vi "Vision Processing.vi"(4 "error in (no error)":errorcluster, 7 "Image Size":T1=enum."320x240") -> ()   [LabVIEW 2016]
doc: "This VI runs in parallel to other tasks. It gets images from the camera, processes them for color or shape and use that information to affect robot behavior."
uses:
  <vilib>/Rock Robotics/WPI/Camera/WPI_CameraImageSize.ctl
  <vilib>/Rock Robotics/WPI/Camera/WPI_CameraWhite Balance Values.ctl
  <vilib>/Rock Robotics/WPI/Camera/WPI_CameraExposure Values.ctl
  <vilib>/Rock Robotics/WPI/Camera/WPI_CameraFrameRate.ctl
  Robot Global Data.vi
  <vilib>/vision/Image Controls.llb/IMAQ Image.ctl
panel:
  in  "Image Size 2":T1=enum."320x240"
  out "x-y":u32
  out "Gear Data":T2
  out "Peg Data":T2
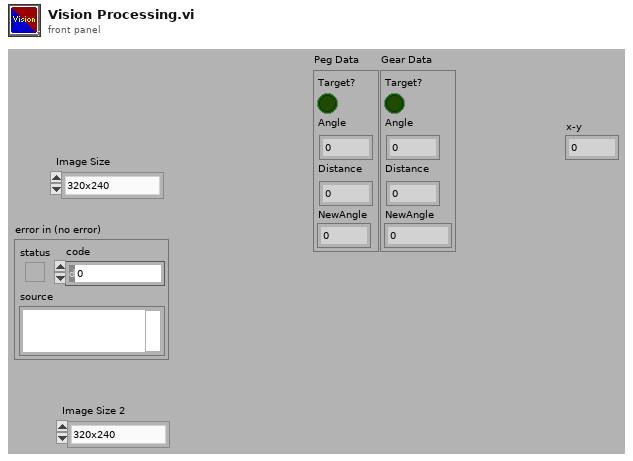
[diagram p1: front panel]
types:
  T1 = typedef "WPI_CameraImageSize.ctl" = enum16{"640x480", "320x240", "160x120", "Custom"}
  T2 = cluster{"Target?":bool, "Angle":dbl, "Distance":dbl, "NewAngle":dbl}
  T3 = typedef "Image Type" = u32
  T4 = typedef "WPI_CameraFrameRate.ctl" = u32
  T5 = typedef "WPI_CameraExposure Values.ctl" = enum16{"Auto", "Flicker-free 50 Hz", "Flicker-free 60 Hz", "Hold current", "Custom"}
  T6 = typedef "WPI_CameraWhite Balance Values.ctl" = enum16{"Auto", "Fixed indoor", "Fixed outdoor 1", "Fixed outdoor 2", "Fixed fluorescent 1", "Fixed fluorescent 2", "Hold current", "Custom"}
  T7 = typedef "IMAQ Image.ctl" = refnum<image>
  T8 = typedef "WPI_CameraDevRef.ctl" = cluster{"Camera Address":string, "CameraStatus":errorcluster}
  T9 = cluster{"Target?":bool, "Angle":dbl, "Distance":dbl}
  T10 = cluster{"Rectangle":cluster{"L":dbl, "T":dbl, "R":dbl, "B":dbl}, "Center":cluster{"X":dbl, "Y":dbl}}
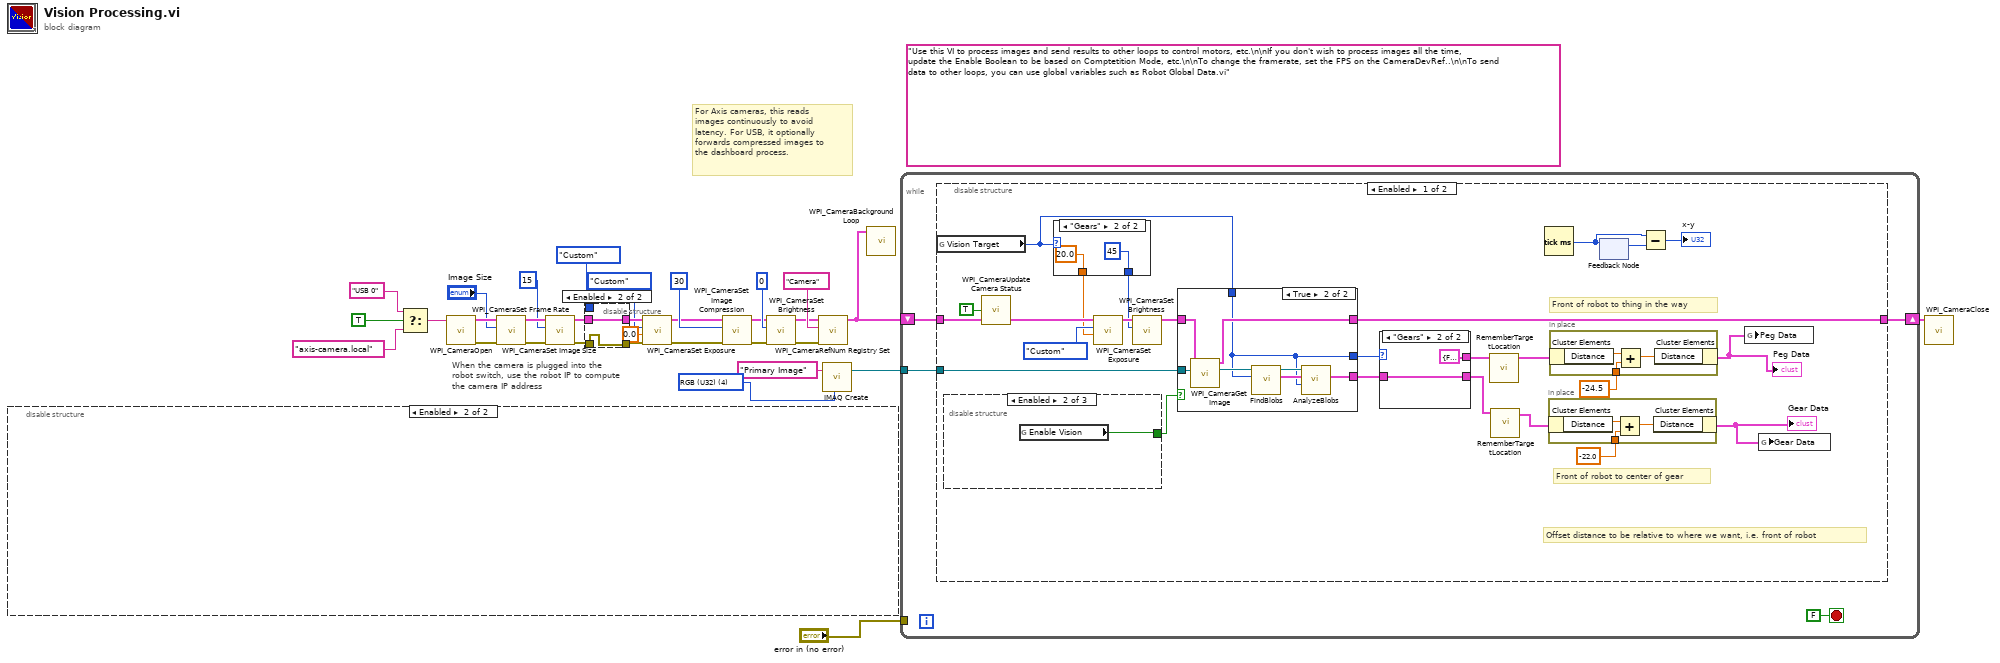
[diagram p0: block diagram]
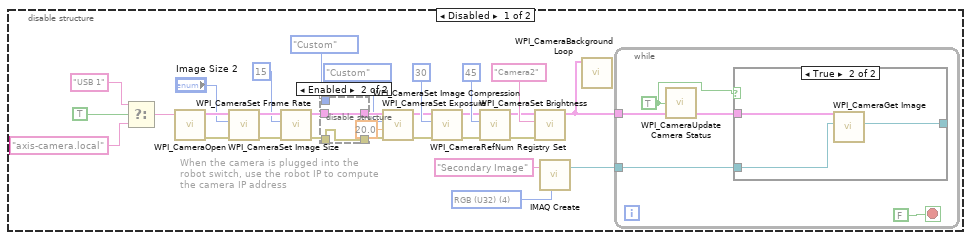
[diagram p2: hidden frame]
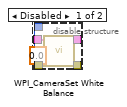
[diagram p3: hidden frame]
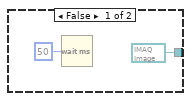
[diagram p4: hidden frame]
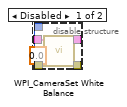
[diagram p5: hidden frame]
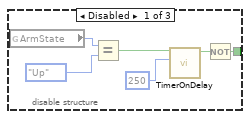
[diagram p6: hidden frame]
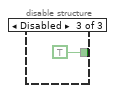
[diagram p7: hidden frame]
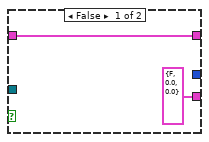
[diagram p8: hidden frame]
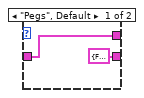
[diagram p9: hidden frame]
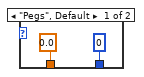
[diagram p10: hidden frame]
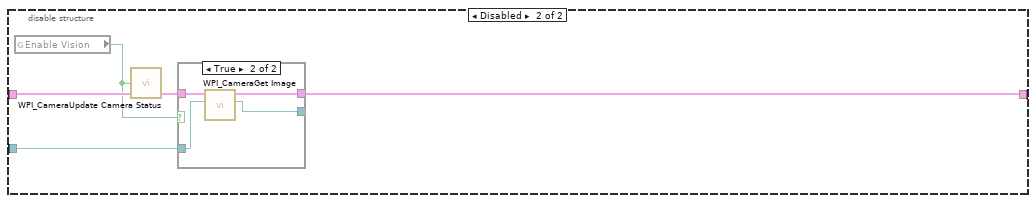
[diagram p11: hidden frame]
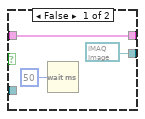
[diagram p12: hidden frame]
diagram:
  w1 = T3 4 items=["Grayscale (U8)", "Grayscale (I16)", "Grayscale (SGL)", "Complex (CSG)", "RGB (U32)", "HSL (U32)", "RGB (U64)"] ("Image Type")
  (unwired) "Use this VI to process images and send results to other loops to control motors, etc.\n\nIf you don't wish to process images all the time, update the Enable Boolean to be based on Comptetition Mode, etc.\n\nTo change the framerate, set the FPS on the CameraDevRef..\n\nTo send data to other loops, you can use global variables such as Robot Global Data.vi"
  # "When the camera is plugged into the\nrobot switch, use the robot IP to compute\nthe camera IP address"
  # "For Axis cameras, this reads\nimages continuously to avoid\nlatency. For USB, it optionally\nforwards compressed images to\nthe dashboard process."
  n1 = disable-structure shown="Enabled" {
    frame Disabled {
      w62 = T3 4 items=["Grayscale (U8)", "Grayscale (I16)", "Grayscale (SGL)", "Complex (CSG)", "RGB (U32)", "HSL (U32)", "RGB (U64)"] ("Image Type")
      # "When the camera is plugged into the\nrobot switch, use the robot IP to compute\nthe camera IP address"
      n2 = Select(t="USB 1" ("format string"), s=TRUE ("dot notation? (F)"), f="axis-camera.local" ("format string")) -> (s? t:f=w37:string)
      n3 = call <vilib>:"WPI_CameraOpen.vi"("Camera Address"=w37) -> ("error out"=w51:errorcluster, "CameraDevRef"=w52:T8)  [unwired: 1 in, 8 out]
      n4 = call <vilib>:"WPI_CameraSet Image Size.vi"("error in (no error)"=w51, "Image Size"="Image Size 2", "CameraDevRef"=w52) -> ("error out"=w50:errorcluster, "CameraDevRef Out"=w53:T8)  [unwired: 1 in, 6 out]
      n5 = call <vilib>:"WPI_CameraSet Frame Rate.vi"("error in (no error)"=w50, "Frame Rate (fps)"=T4 15, "CameraDevRef"=w53) -> ("error out"=w49:errorcluster, "CameraDevRef Out"=w55:T8)  [unwired: 7 out]
      n6 = disable-structure shown="Enabled" {
        disable-tunnel: w55 -> [w68 w70]
        disable-tunnel: [w67 w70] -> w54
        disable-tunnel: w49 -> [w66 w69]
        disable-tunnel: [w65 w69] -> w48
        disable-tunnel: WPI_CameraWhite_Balance_Values."Custom" ("White Balance") -> [w64 _]
        frame Disabled {
          n7 = call <vilib>:"WPI_CameraSet White Balance.vi"("error in (no error)"=w66, "Color Temp (K)"=0.0, "White Balance"=w64, "CameraDevRef"=w68) -> ("error out"=w65:errorcluster, "CameraDevRef Out"=w67:T8)  [unwired: 6 out]
        }
        frame Enabled {
        }
      }
      n8 = call <vilib>:"WPI_CameraSet Exposure.vi"("error in (no error)"=w48, "Exposure (%)"=20.0, "Exposure"=WPI_CameraExposure_Values."Custom", "CameraDevRef"=w54) -> ("error out"=w47:errorcluster, "CameraDevRef Out"=w57:T8)  [unwired: 6 out]
      n9 = call <vilib>:"WPI_CameraSet Image Compression.vi"("error in (no error)"=w47, "Compression"=30, "CameraDevRef"=w57) -> ("error out"=w46:errorcluster, "CameraDevRef Out"=w56:T8)  [unwired: 7 out]
      n10 = call <vilib>:"WPI_CameraSet Brightness.vi"("error in (no error)"=w46, "Brightness"=45, "CameraDevRef"=w56) -> ("error out"=w44:errorcluster, "CameraDevRef Out"=w45:T8)  [unwired: 7 out]
      n11 = call <vilib>:"WPI_CameraRefNum Registry Set.vi"("error in (no error)"=w44, "refnum name"="Camera2", "CameraDevRef"=w45) -> ("CameraDevRef"=w34:T8)  [unwired: 1 in, 7 out]
      n12 = call "IMAQ Create"("Image Name"="Secondary Image", "Image Type"=w62) -> ("New Image"=w33:T7)  [unwired: 2 in, 2 out]
      n13 = call <vilib>:"WPI_CameraBackground Loop.vi"("CameraDevRef"=w34) -> ()  [unwired: 11 in]
      n14 = while {
        tunnel: w34 -> [w75]
        tunnel: w33 -> [w72]
        stop <- FALSE stop-if-true
        w71 = TRUE ("Enable Vision")
        n15 = call <vilib>:"WPI_CameraUpdate Camera Status.vi"("CameraDevRef In"=w75, "Enable Vision"=w71) -> ("CameraDevRef Out"=w73:T8)  [unwired: 3 in]
        n16 = case shown="True" w71 {
          tunnel: w73 -> [_ w78]
          tunnel: w72 -> [_ w80]
          tunnel: [T7 refnum ("Image Out") w79] -> _
          frame False {
            n17 = Wait (ms)(milliseconds to wait=u32 50) -> ()  [unwired: 1 out]
          }
          frame True {
            n18 = call <vilib>:"WPI_CameraGet Image.vi"("Image"=w80, "CameraDevRef"=w78) -> ("Image Out"=w79:T7)  [unwired: 1 in, 8 out]
          }
        }
      }
    }
    frame Enabled {
    }
  }
  n19 = Select(t="USB 0" ("format string"), s=TRUE ("dot notation? (F)"), f="axis-camera.local" ("format string")) -> (s? t:f=w4:string)
  n20 = call <vilib>:"WPI_CameraOpen.vi"("Camera Address"=w4) -> ("error out"=w21:errorcluster, "CameraDevRef"=w22:T8)  [unwired: 1 in, 8 out]
  n21 = call <vilib>:"WPI_CameraSet Image Size.vi"("error in (no error)"=w21, "Image Size"="Image Size", "CameraDevRef"=w22) -> ("error out"=w20:errorcluster, "CameraDevRef Out"=w23:T8)  [unwired: 1 in, 6 out]
  n22 = call <vilib>:"WPI_CameraSet Frame Rate.vi"("error in (no error)"=w20, "Frame Rate (fps)"=T4 15, "CameraDevRef"=w23) -> ("error out"=w19:errorcluster, "CameraDevRef Out"=w25:T8)  [unwired: 7 out]
  n23 = disable-structure shown="Enabled" {
    disable-tunnel: w25 -> [w86 w88]
    disable-tunnel: [w85 w88] -> w24
    disable-tunnel: w19 -> [w84 w87]
    disable-tunnel: [w83 w87] -> w18
    disable-tunnel: WPI_CameraWhite_Balance_Values."Custom" ("White Balance") -> [w82 _]
    frame Disabled {
      n24 = call <vilib>:"WPI_CameraSet White Balance.vi"("error in (no error)"=w84, "Color Temp (K)"=0.0, "White Balance"=w82, "CameraDevRef"=w86) -> ("error out"=w83:errorcluster, "CameraDevRef Out"=w85:T8)  [unwired: 6 out]
    }
    frame Enabled {
    }
  }
  n25 = call <vilib>:"WPI_CameraSet Exposure.vi"("error in (no error)"=w18, "Exposure (%)"=0.0, "Exposure"=WPI_CameraExposure_Values."Custom", "CameraDevRef"=w24) -> ("error out"=w17:errorcluster, "CameraDevRef Out"=w27:T8)  [unwired: 6 out]
  n26 = call <vilib>:"WPI_CameraSet Image Compression.vi"("error in (no error)"=w17, "Compression"=30, "CameraDevRef"=w27) -> ("error out"=w16:errorcluster, "CameraDevRef Out"=w26:T8)  [unwired: 7 out]
  n27 = call <vilib>:"WPI_CameraSet Brightness.vi"("error in (no error)"=w16, "Brightness"=0, "CameraDevRef"=w26) -> ("error out"=w14:errorcluster, "CameraDevRef Out"=w15:T8)  [unwired: 7 out]
  n28 = call <vilib>:"WPI_CameraRefNum Registry Set.vi"("error in (no error)"=w14, "refnum name"="Camera", "CameraDevRef"=w15) -> ("CameraDevRef"=w10:T8)  [unwired: 1 in, 7 out]
  n29 = call "IMAQ Create"("Image Name"="Primary Image", "Image Type"=w1) -> ("New Image"=w31:T7)  [unwired: 2 in, 2 out]
  n30 = call <vilib>:"WPI_CameraBackground Loop.vi"("CameraDevRef"=w10) -> ()  [unwired: 11 in]
  n31 = while {
    shift-right: [w91] -> w8
    shift-left: w10 -> [w89]
    tunnel: w31 -> [w90]
    tunnel: "error in (no error)" -> [_]
    stop <- FALSE stop-if-true
    n32 = disable-structure shown="Enabled" {
      disable-tunnel: [w117 w150] -> w91
      disable-tunnel: w90 -> [w116 w151]
      disable-tunnel: w89 -> [w115 w154]
      frame Enabled {
        # "Front of robot to center of gear"
        # "Front of robot to thing in the way"
        # "Offset distance to be relative to where we want, i.e. front of robot"
        n33 = global read "Robot Global Data.vi" "Vision Target"() -> (w113:enum16{"Pegs", "Gears"})
        n34 = disable-structure shown="Enabled" {
          disable-tunnel: [w119 w124 TRUE] -> w93
          frame Disabled {
            n35 = global read "Robot Global Data.vi" "ArmState"() -> (w123:enum16{"Up", "Down"})
            n36 = Equal?(x=w123, y=enum16{"Up", "Down"}."Up") -> (x = y?=w118:bool)
            n37 = call "TimerOnDelay.vi"("Time Limit"=u32 250, "Input"=w118) -> ("Output"=w120:bool)  [unwired: 9 in]
            n38 = Not(x=w120) -> (.not. x?=w119:bool)
          }
          frame Enabled {
            n39 = global read "Robot Global Data.vi" "Enable Vision"() -> (w124:bool)
          }
          frame Disabled {
          }
        }
        n40 = call <vilib>:"WPI_CameraUpdate Camera Status.vi"("CameraDevRef In"=w115, "Enable Vision"=TRUE) -> ("CameraDevRef Out"=w114:T8)  [unwired: 3 in]
        n41 = case shown="\"Gears\"" w113 {
          tunnel: [0.0 ("Exposure (%)") 20.0 ("Exposure (%)")] -> w109
          tunnel: [0 ("Compression") 45 ("Compression")] -> w108
          frame "Pegs", Default {
          }
          frame "Gears" {
          }
        }
        n42 = call <vilib>:"WPI_CameraSet Exposure.vi"("Exposure (%)"=w109, "Exposure"=WPI_CameraExposure_Values."Custom", "CameraDevRef"=w114) -> ("CameraDevRef Out"=w112:T8)  [unwired: 1 in, 7 out]
        n43 = call <vilib>:"WPI_CameraSet Brightness.vi"("Brightness"=w108, "CameraDevRef"=w112) -> ("CameraDevRef Out"=w111:T8)  [unwired: 1 in, 8 out]
        n44 = case shown="True" w93 {
          tunnel: w116 -> [_ w135]
          tunnel: [w127 w134] -> w117
          tunnel: w111 -> [w127 w133]
          tunnel: w113 -> [_ w128]
          tunnel: [T9 {"Target?"=FALSE, "Angle"=0.0, "Distance"=0.0} ("Target Data") w131] -> w107
          tunnel: [_ w128] -> w95
          frame False {
          }
          frame True {
            n45 = call <vilib>:"WPI_CameraGet Image.vi"("Image"=w135, "CameraDevRef"=w133) -> ("Image Out"=w130:T7, "CameraDevRef Out"=w134:T8)  [unwired: 1 in, 7 out]
            n46 = call "FindBlobs.vi"("Vision Target"=w128, "Image In"=w130) -> ("Blob Data"=w129:T10, "Image Out"=w132:T7)  [unwired: 8 in]
            n47 = call "AnalyzeBlobs.vi"("Vision Target"=w128, "Blob Data"=w129, "Image In"=w132) -> ("Target Data"=w131:T9)  [unwired: 7 in, 1 out]
          }
        }
        n48 = case shown="\"Gears\"" w95 {
          tunnel: w107 -> [w142 w145]
          tunnel: [T9 {"Target?"=FALSE, "Angle"=0.0, "Distance"=inf} ("Target Data") w145] -> w106
          tunnel: [w142 T9 {"Target?"=FALSE, "Angle"=0.0, "Distance"=inf} ("Target Data")] -> w105
          frame "Pegs", Default {
          }
          frame "Gears" {
          }
        }
        n49 = call "RememberTargetLocation.vi"("Target Data"=w105) -> ("Peg Data"=w104:T2)  [unwired: 10 in]
        n50 = call "RememberTargetLocation.vi"("Target Data"=w106) -> ("Peg Data"=w100:T2)  [unwired: 10 in]
        n51 = Tick Count (ms)() -> (millisecond timer value=w97:u32)
        n52 = in-place {
          in-place-border: -22.0 -> [w137]
          n53 = in-place-cluster #1(w100) -> ("Distance"=w138:dbl)
          n54 = Add(x=w138, y=w137) -> (x+y=w136:dbl)
          n55 = in-place-cluster #1("Distance"=w136) -> (w99:T2)
        }
        "Gear Data" <- w99
        n56 = in-place {
          in-place-border: -24.5 -> [w140]
          n57 = in-place-cluster #2(w104) -> ("Distance"=w141:dbl)
          n58 = Add(x=w141, y=w140) -> (x+y=w139:dbl)
          n59 = in-place-cluster #2("Distance"=w139) -> (w103:T2)
        }
        "Peg Data" <- w103
        n60 = feedback #3() -> (w96:u32)  [unwired: 1 in]
        n61 = feedback-in #3(w97) -> ()
        n62 = Subtract(x=w97, y=w96) -> (x-y=→"x-y":u32)
        n63 = global write "Robot Global Data.vi" "Peg Data"(w103) -> ()
        n64 = global write "Robot Global Data.vi" "Gear Data"(w99) -> ()
      }
      frame Disabled {
        n65 = global read "Robot Global Data.vi" "Enable Vision"() -> (w153:bool)
        n66 = call <vilib>:"WPI_CameraUpdate Camera Status.vi"("CameraDevRef In"=w154, "Enable Vision"=w153) -> ("CameraDevRef Out"=w152:T8)  [unwired: 3 in]
        n67 = case shown="True" w153 {
          tunnel: w152 -> [w155 w161]
          tunnel: [T7 refnum ("Image Out") w158] -> _
          tunnel: w151 -> [_ w160]
          tunnel: [w155 w159] -> w150
          frame False {
            n68 = Wait (ms)(milliseconds to wait=u32 50) -> ()  [unwired: 1 out]
          }
          frame True {
            n69 = call <vilib>:"WPI_CameraGet Image.vi"("Image"=w160, "CameraDevRef"=w161) -> ("Image Out"=w158:T7, "CameraDevRef Out"=w159:T8)  [unwired: 1 in, 7 out]
          }
        }
      }
    }
  }
  n70 = call <vilib>:"WPI_CameraClose.vi"("CameraDevRef"=w8) -> ()  [unwired: 1 in, 10 out]
